vi "Fahrenheit.vi"(3 "C":dbl) -> (1 "F":dbl)   [LabVIEW 2014]
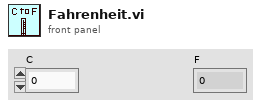
[diagram p1: front panel]
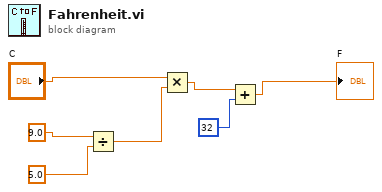
[diagram p0: block diagram]
diagram:
  n1 = Divide(x=9.0, y=5.0) -> (x/y=w6:dbl)
  n2 = Multiply(x="C", y=w6) -> (x*y=w3:dbl)
  n3 = Add(x=w3, y=32) -> (x+y=→"F":dbl)
